vi "_counter.vi"() -> (2 "out_count":string)   [LabVIEW 2023]
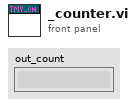
[diagram p1: front panel]
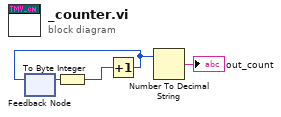
[diagram p0: block diagram]
diagram:
  n1 = feedback #1() -> (w4:i8)  [unwired: 1 in]
  n2 = To Byte Integer(number=w4) -> (8bit integer=w2:i8)
  n3 = Increment(x=w2) -> (x+1=w3:i8)
  n4 = feedback-in #1(w3) -> ()
  n5 = Number To Decimal String(number=w3) -> (decimal integer string=→"out_count":string)  [unwired: 1 in]
